vi "Remove First and Last Characters.vi"(11 "Quoted String":string) -> (3 "String":string)   [LabVIEW 2015, in "RTSequenceVIs.lvlib"]
doc: "Removes the first and last character from the string."
uses:
  RTSequenceVIs.lvlib
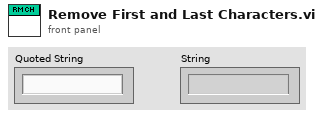
[diagram p1: front panel]
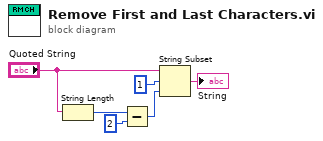
[diagram p0: block diagram]
diagram:
  n1 = String Length(string="Quoted String") -> (length=w3:i32)
  n2 = Subtract(x=w3, y=2) -> (x-y=w5:i32)
  n3 = String Subset(string="Quoted String", offset (0)=1, length (rest)=w5) -> (substring=→"String":string)
